vi "Seq Graph.vi"(8 "Error In":errorcluster, 10 "Iteration":i32, 11 "Sequence":T1(array[cluster])=[{"Duration"=10, "Value"=100, "Name"="Step1"}, {"Duration"=60, "Value"=150, "Name"="Step2"}, {"Duration"=120, "Value"=50, "Name"="Step3"}] {"Duration" format="%<%H:%M:%S>t"}) -> (0 "Error Out":errorcluster, 3 "Waveform":u32[](graph))   [LabVIEW 2019, in "Platform.lvlib" / "Platform.lvclass"]
uses:
  Platform.lvclass
panel:
  # "Step"
  # "Duration"
  # "Value"
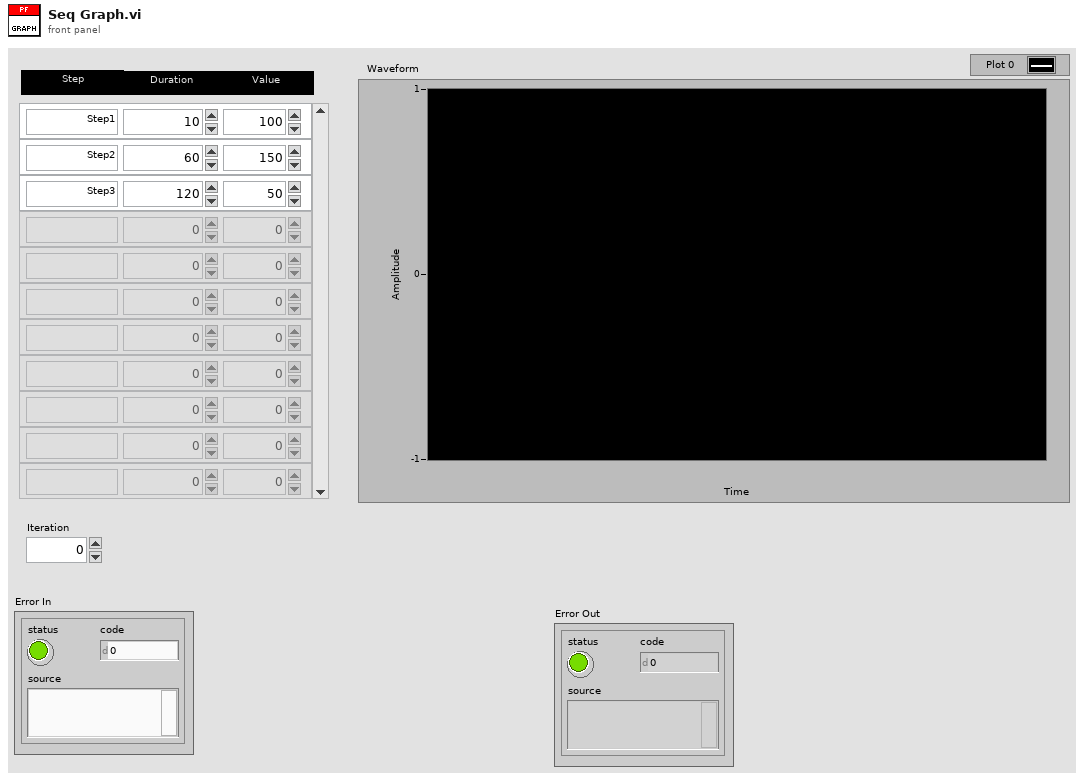
[diagram p1: front panel]
types:
  T1 = cluster{"Duration":i32, "Value":u32, "Name":string}[]
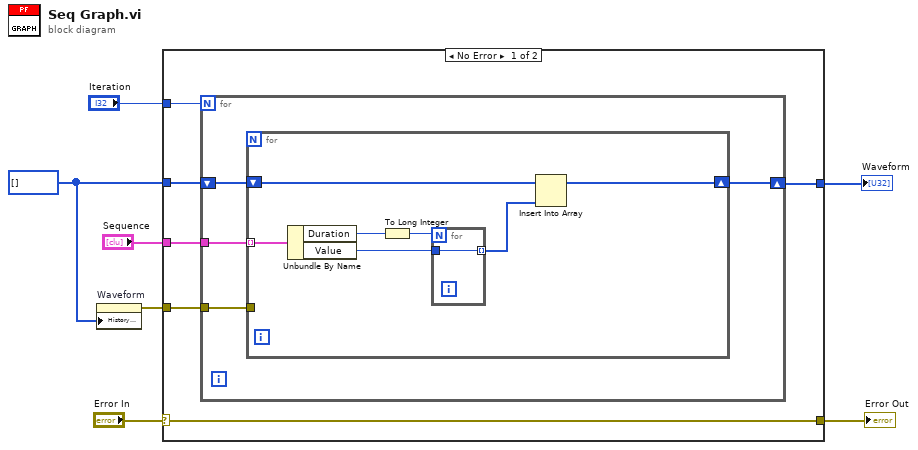
[diagram p0: block diagram]
diagram:
  w2 = u32[] []
  n1 = property on="Waveform" class="WFChart (strict)"("History Data"=w2) -> (error out=w6:errorcluster)  [unwired: 2 in, 1 out]
  n2 = case shown="No Error" "Error In" {
    selector: "Error In" -> [w10 w27]
    tunnel: "Sequence" -> [w13 _]
    tunnel: w6 -> [w12 _]
    tunnel: w2 -> [w11 w26]
    tunnel: [w10 w27] -> w4
    tunnel: "Iteration" -> [w9 _]
    tunnel: [w8 w26] -> w1
    frame No Error {
      n3 = for {
        N: w9 -> [_]
        tunnel: w13 -> [w17]
        tunnel: w12 -> [w16]
        shift-right: [w14] -> w8
        shift-left: w11 -> [w15]
        n4 = for {
          tunnel: w17 -> [w24] mode=indexing
          tunnel: w16 -> [_]
          shift-right: [w18] -> w14
          shift-left: w15 -> [w23]
          n5 = Unbundle By Name(w24) -> ("Duration"=w22:i32, "Value"=w21:u32)
          n6 = To Long Integer(number=w22) -> (32bit integer=w20:i32)
          n7 = for {
            N: w20 -> [_]
            tunnel: w21 -> [w25]
            tunnel: [w25] -> w19 mode=indexing
          }
          n8 = Insert Into Array(array=w23, new element=w19) -> (w18:u32[])  [unwired: 1 in]
        }
      }
    }
    frame Error {
    }
  }
  "Error Out" <- w4
  "Waveform" <- w1
